vi "Offset Yaw.vi"(9 "Sensor Yaw":dbl, 10 "Trigger offset":bool) -> (3 "Yaw with offset":dbl)   [LabVIEW 2016]
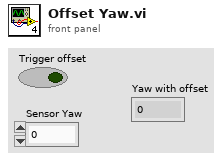
[diagram p1: front panel]
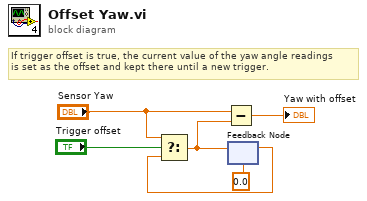
[diagram p0: block diagram]
diagram:
  # "If trigger offset is true, the current value of the yaw angle readings\nis set as the offset and kept there until a new trigger."
  n1 = feedback #1(0.0) -> (w4:dbl)
  n2 = Select(t="Sensor Yaw", s="Trigger offset", f=w4) -> (s? t:f=w1:dbl)
  n3 = Subtract(x="Sensor Yaw", y=w1) -> (x-y=→"Yaw with offset":dbl)
  n4 = feedback-in #1(w1) -> ()
